vi "Get Owning Custom Device.vi"(8 "error in":errorcluster, 11 "item":T1 format="%.0x") -> (0 "error out":errorcluster, 2 "owning custom device":T1=18446744073709551615 format="%.0x", 3 "item out":T1 format="%.0x")   [LabVIEW 2020, in "Ballard MIL-STD-1553 System Explorer.lvlib" / "Implementation.lvlib" / "System Explorer Dispatcher.lvclass"]
uses:
  System Explorer Dispatcher.lvclass
  <vilib>/NI VeriStand/Custom Device API/Custom Device Item Ref.ctl
  Scripting/Constants.vi
  Scripting/Ballard MIL-STD-1553 Scripting.lvlib
  <vilib>/NI VeriStand/Custom Device Tools/Custom Device Utility Library/Custom Device Utility Library.lvlib
  <vilib>/NI VeriStand/Custom Device Tools/Custom Device Utility Library/Search Direction.ctl
  <vilib>/NI VeriStand/Custom Device Tools/Custom Device Utility Library/NI VeriStand - Search for Item by GUID.vi
  <vilib>/NI VeriStand/Custom Device API/Custom Device API.lvlib
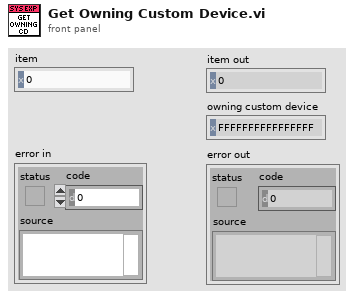
[diagram p1: front panel]
types:
  T1 = typedef "Custom Device API.lvlib/Custom Device Item Ref.ctl" = u64
  T2 = typedef "Custom Device Utility Library.lvlib/Search Direction.ctl" = enum16{"Down", "Up"}
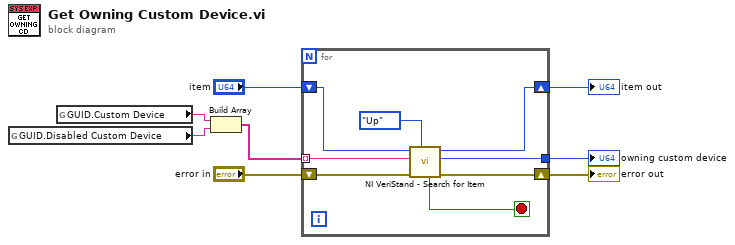
[diagram p0: block diagram]
diagram:
  n1 = global read "Constants.vi" "GUID.Disabled Custom Device"() -> (w8:string)
  n2 = global read "Constants.vi" "GUID.Custom Device"() -> (w7:string)
  n3 = Build Array(w7, w8) -> (w2:string[])
  n4 = for {
    shift-right: [w12] -> w3
    shift-left: "error in" -> [w16]
    shift-right: [w13] -> w1
    shift-left: "item" -> [w14]
    tunnel: [w11] -> w4
    tunnel: w2 -> [w9] mode=indexing
    stop <- w10 stop-if-true
    n5 = call-poly <vilib>:"NI VeriStand - Search for Item.vi"("Direction (Down)"=Search_Direction."Up", "error in"=w16, "Item GUID"=w9, "Section Ref in"=w14) -> ("error out"=w12:errorcluster, "Item Ref"=w11:T1, "Section Ref out"=w13:T1, "Found"=w10:bool)  [unwired: 4 in]
  }
  "item out" <- w1
  "error out" <- w3
  "owning custom device" <- w4
